vi "extrapolate samples.vi"(1 "ramp array in":u32[](array[numeric]), 2 "new sample number":i32) -> (0 "extrapolated array out":u32[](array[numeric]))   [LabVIEW 2010, in "ColorOverlay.lvclass"]
uses:
  ColorOverlay.lvclass
  <vilib>/gmath/NI_Gmath.lvlib
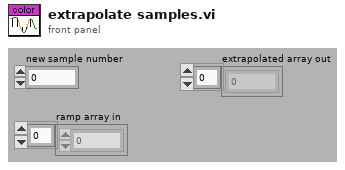
[diagram p1: front panel]
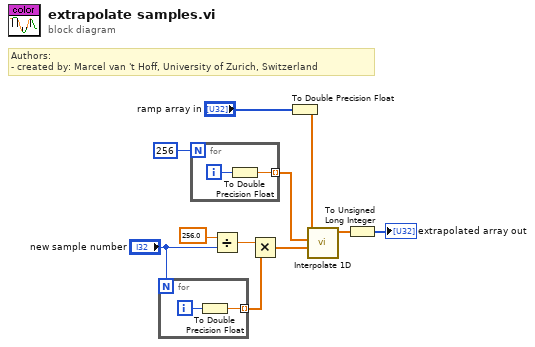
[diagram p0: block diagram]
diagram:
  # "Authors: \n- created by: Marcel van 't Hoff, University of Zurich, Switzerland"
  n1 = for {
    N: "new sample number" -> [_]
    tunnel: [w12] -> w2 mode=indexing
    i -> [w13]
    n2 = To Double Precision Float(number=w13) -> (double precision float=w12:dbl)
  }
  n3 = for {
    N: 256 -> [_]
    tunnel: [w14] -> w4 mode=indexing
    i -> [w15]
    n4 = To Double Precision Float(number=w15) -> (double precision float=w14:dbl)
  }
  n5 = Divide(x=256.0, y="new sample number") -> (x/y=w7:dbl)
  n6 = Multiply(x=w7, y=w2) -> (x*y=w8:dbl[])
  n7 = To Double Precision Float(number="ramp array in") -> (double precision float=w1:dbl[])
  n8 = call <vilib>:"Interpolate 1D.vi"("xi"=w8, "X"=w4, "Y"=w1) -> ("yi"=w10:dbl[])  [unwired: 6 in, 2 out]
  n9 = To Unsigned Long Integer(number=w10) -> (unsigned 32bit integer=→"extrapolated array out":u32[])
